vi "microFPGA_laser_mode_addr_0_ctrl.vi"(0 "VISA resource name":refnum<visa-resource-name>, 1 "laser channel":u16(ring)=3 items=["channel No 0", "channel No 1", "channel No 2", "channel No 3", "channel No 4", "channel No 5"], 2 "write or read":u16(ring) items=["read", "write"], 7 "laser mode write":u16(ring) items=["OFF", "ON", "RISING", "FALLING", "CAMERA"], 11 "error in (no error)":errorcluster) -> (4 "VISA resource name out":refnum<visa-resource-name>, 6 "laser mode read":u32(ring) items=["OFF", "ON", "RISING", "FALLING", "CAMERA"], 8 "value write confirm":bool, 10 "abort_wrong_input":bool, 15 "error out":errorcluster)   [LabVIEW 2016]
panel:
  out "mode read string answer":string
  out "mode read string":string
  out "mode write string":string
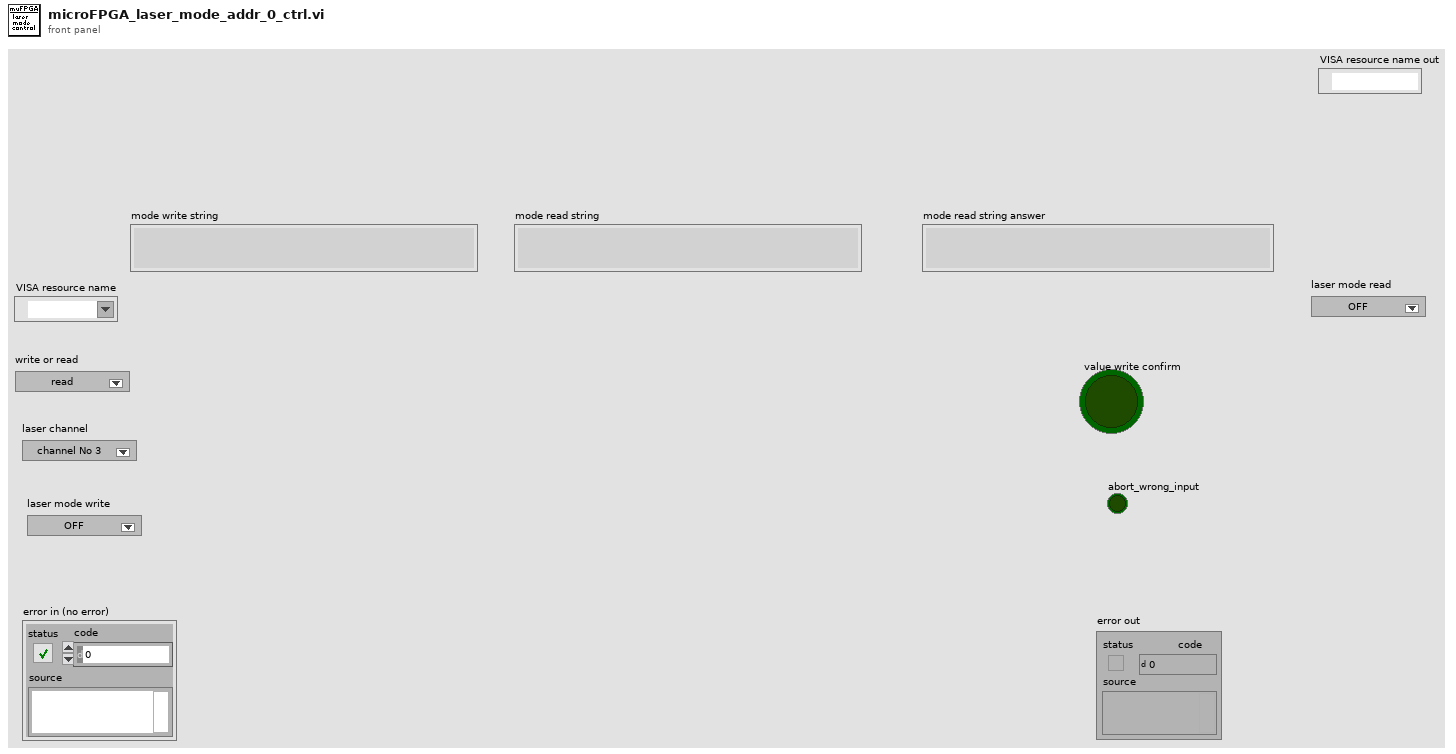
[diagram p1: front panel]
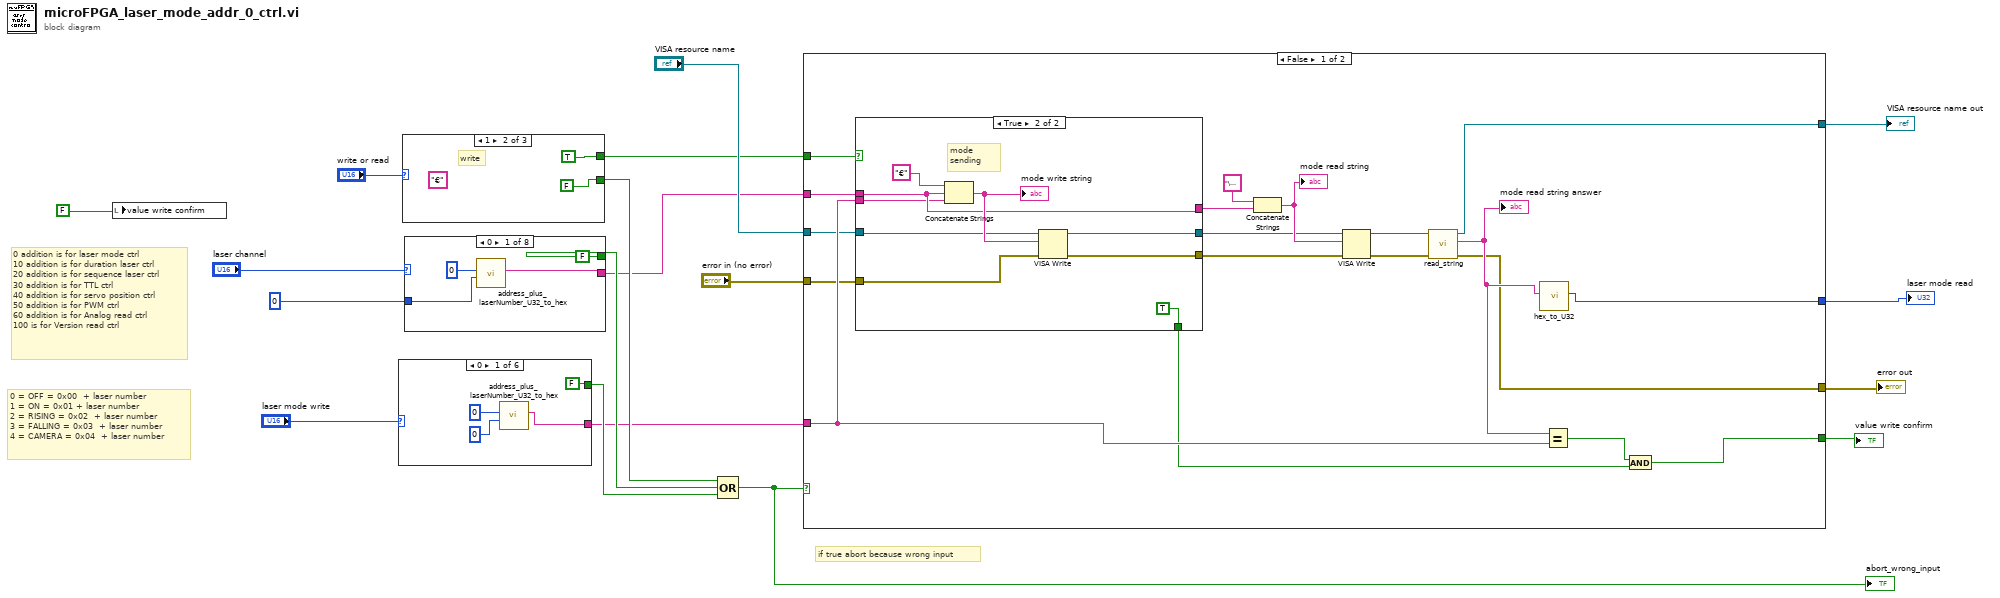
[diagram p0: block diagram]
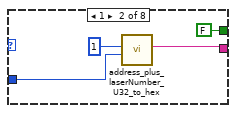
[diagram p2: hidden frame]
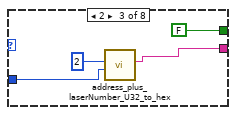
[diagram p3: hidden frame]
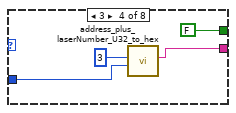
[diagram p4: hidden frame]
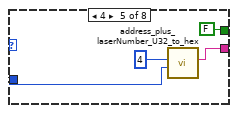
[diagram p5: hidden frame]
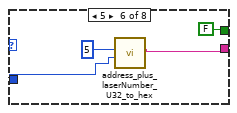
[diagram p6: hidden frame]
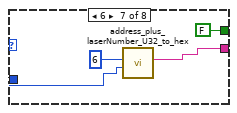
[diagram p7: hidden frame]
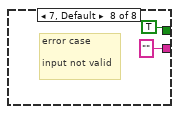
[diagram p8: hidden frame]
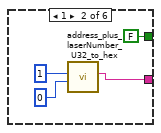
[diagram p9: hidden frame]
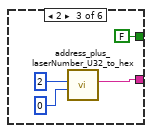
[diagram p10: hidden frame]
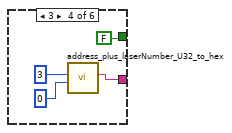
[diagram p11: hidden frame]
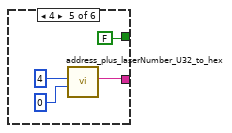
[diagram p12: hidden frame]
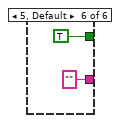
[diagram p13: hidden frame]
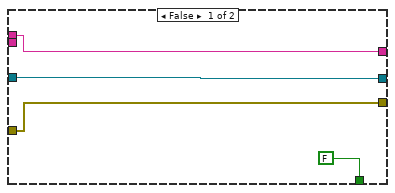
[diagram p14: hidden frame]
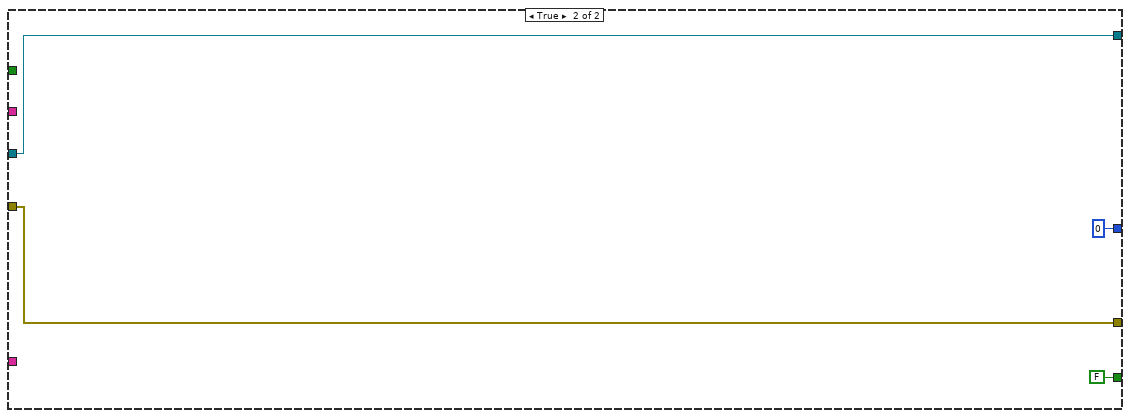
[diagram p15: hidden frame]
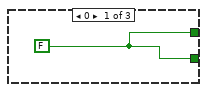
[diagram p16: hidden frame]
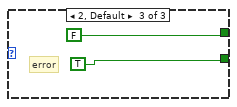
[diagram p17: hidden frame]
diagram:
  # "0 addition is for laser mode ctrl\n10 addition is for duration laser ctrl\n20 addition is for sequence laser ctrl\n30 addition is for TTL ctrl\n40 addition is for servo position ctrl\n50 addition is for PWM ctrl\n60 addition is for Analog read ctrl\n100 is for Version read ctrl"
  # "0 = OFF = 0x00  + laser number\n1 = ON = 0x01 + laser number\n2 = RISING = 0x02  + laser number\n3 = FALLING = 0x03  + laser number\n4 = CAMERA = 0x04  + laser number"
  # "if true abort because wrong input"
  n1 = local write "value write confirm"(FALSE ("value confirm")) -> ()
  n2 = case shown="0" "laser mode write" {
    tunnel: [w19 w24 w28 w32 w36 "" ("string 5")] -> w2
    tunnel: [FALSE FALSE FALSE FALSE FALSE TRUE] -> w8
    frame 0 {
      n3 = call "address_plus_laserNumber_U32_to_hex.vi"("adress offset"=u32 0, "y 3"=u32 0) -> ("string 5"=w19:string)  [unwired: 8 in]
    }
    frame 1 {
      n4 = call "address_plus_laserNumber_U32_to_hex.vi"("adress offset"=u32 0, "y 3"=u32 1) -> ("string 5"=w24:string)  [unwired: 8 in]
    }
    frame 2 {
      n5 = call "address_plus_laserNumber_U32_to_hex.vi"("adress offset"=u32 0, "y 3"=u32 2) -> ("string 5"=w28:string)  [unwired: 8 in]
    }
    frame 3 {
      n6 = call "address_plus_laserNumber_U32_to_hex.vi"("adress offset"=u32 0, "y 3"=u32 3) -> ("string 5"=w32:string)  [unwired: 8 in]
    }
    frame 4 {
      n7 = call "address_plus_laserNumber_U32_to_hex.vi"("adress offset"=u32 0, "y 3"=u32 4) -> ("string 5"=w36:string)  [unwired: 8 in]
    }
    frame 5, Default {
    }
  }
  n8 = case shown="1" "write or read" {
    tunnel: [w41 TRUE FALSE] -> w16
    tunnel: [w41 FALSE TRUE] -> w14
    frame 0 {
      w41 = FALSE
    }
    frame 1 {
      (unwired) "€" ("hex")
      # "write"
    }
    frame 2, Default {
      # "error"
    }
  }
  n9 = case shown="0" "laser channel" {
    tunnel: [w47 w51 w55 w59 w63 w67 w71 "" ("string 5")] -> w3
    tunnel: [FALSE FALSE FALSE FALSE FALSE FALSE FALSE TRUE] -> w4
    tunnel: u32 0 ("adress offset") -> [w46 w50 w54 w58 w62 w66 w70 _]
    frame 0 {
      n10 = call "address_plus_laserNumber_U32_to_hex.vi"("adress offset"=w46, "y 3"=u32 0) -> ("string 5"=w47:string)  [unwired: 8 in]
    }
    frame 1 {
      n11 = call "address_plus_laserNumber_U32_to_hex.vi"("adress offset"=w50, "y 3"=u32 1) -> ("string 5"=w51:string)  [unwired: 8 in]
    }
    frame 2 {
      n12 = call "address_plus_laserNumber_U32_to_hex.vi"("adress offset"=w54, "y 3"=u32 2) -> ("string 5"=w55:string)  [unwired: 8 in]
    }
    frame 3 {
      n13 = call "address_plus_laserNumber_U32_to_hex.vi"("adress offset"=w58, "y 3"=u32 3) -> ("string 5"=w59:string)  [unwired: 8 in]
    }
    frame 4 {
      n14 = call "address_plus_laserNumber_U32_to_hex.vi"("adress offset"=w62, "y 3"=u32 4) -> ("string 5"=w63:string)  [unwired: 8 in]
    }
    frame 5 {
      n15 = call "address_plus_laserNumber_U32_to_hex.vi"("adress offset"=w66, "y 3"=u32 5) -> ("string 5"=w67:string)  [unwired: 8 in]
    }
    frame 6 {
      n16 = call "address_plus_laserNumber_U32_to_hex.vi"("adress offset"=w70, "y 3"=u32 6) -> ("string 5"=w71:string)  [unwired: 8 in]
    }
    frame 7, Default {
      # "error case\n\ninput not valid"
    }
  }
  n17 = Compound Arithmetic op=OR(w14, w4, w8) -> (w12:bool)
  "abort_wrong_input" <- w12
  n18 = case shown="False" w12 {
    tunnel: "VISA resource name" -> [w77 w109]
    tunnel: w3 -> [w92 _]
    tunnel: w16 -> [w86 _]
    tunnel: w2 -> [w84 _]
    tunnel: [w83 u32 0 ("U32")] -> w7
    tunnel: [w78 FALSE] -> w13
    tunnel: [w82 w109] -> w11
    tunnel: [w81 w108] -> w10
    tunnel: "error in (no error)" -> [w76 w108]
    frame False {
      n19 = case shown="True" w86 {
        tunnel: w92 -> [w98 w105]
        tunnel: [w98 w105] -> w93
        tunnel: w84 -> [_ w104]
        tunnel: [w96 w103] -> w88
        tunnel: [w95 w102] -> w87
        tunnel: [FALSE TRUE] -> w80
        tunnel: w77 -> [w96 w100]
        tunnel: w76 -> [w95 w99]
        frame False {
        }
        frame True {
          # "mode \nsending"
          n20 = Concatenate Strings("€" ("string"), w105, w104) -> (w106:string)
          "mode write string" <- w106
          n21 = VISA Write(VISA resource name=w100, write buffer=w106, error in (no error)=w99) -> (VISA resource name out=w103:refnum<visa-resource-name>, error out=w102:errorcluster)  [unwired: 1 out]
        }
      }
      n22 = Concatenate Strings("\u0000" ("string"), w93) -> (w91:string)
      "mode read string" <- w91
      n23 = VISA Write(VISA resource name=w88, write buffer=w91, error in (no error)=w87) -> (VISA resource name out=w90:refnum<visa-resource-name>, error out=w89:errorcluster)  [unwired: 1 out]
      n24 = call "read_string.vi"("error in"=w89, "VISA resource name"=w90) -> ("error out"=w81:errorcluster, "read buffer"=w85:string, "VISA resource name out"=w82:refnum<visa-resource-name>)  [unwired: 7 in]
      "mode read string answer" <- w85
      n25 = call "hex_to_U32.vi"("hex"=w85) -> ("U32"=w83:u32)  [unwired: 9 in]
      n26 = Equal?(x=w85, y=w84) -> (x = y?=w79:bool)
      n27 = And(x=w79, y=w80) -> (x .and. y?=w78:bool)
    }
    frame True {
    }
  }
  "value write confirm" <- w13
  "VISA resource name out" <- w11
  "error out" <- w10
  "laser mode read" <- w7
